vi "PH_Countdown-Counter.Calc Remaining Time.vi"(0 "i ref in":refnum<vi>, 5 "error in":errorcluster) -> (14 "i ref out":refnum<vi>, 17 "remaining Time [s]":dbl, 19 "error out":errorcluster)   [LabVIEW 2014, in "PH_Countdown-Counter.lvlib"]
uses:
  PH_Countdown-Counter.lvlib
  PH_Basics/PH_PP_Common/PH_PP_Common.PUs.ctl
  PH_Basics/PH_PP_Common/PH_PP_Common.Trigger Tags.ctl
  PH_Basics/PH_Common/PH_Common.lvlib
  CSlibraries-extern/DimLVEvent/LVDimInterface/LVDimInterface.lvlib
  PH_Basics/PH_PP_Common/PH_PP_Common.lvlib
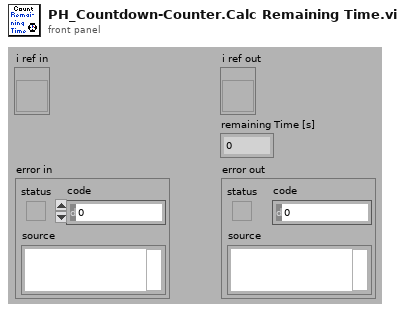
[diagram p1: front panel]
types:
  T1 = typedef "PH_Countdown-Counter.lvlib/PH_Countdown-Counter.i attribute.ctl" = cluster{"Machine Time":cluster{"Tag":string, "Wating Time [s]":dbl, "not linked?":bool}[], "Last Shot":cluster{"Tag":string, "Shot Time [s]":timestamp, "not linked?":bool}[], "Time since last Shot?":bool, "Calculation":cluster{"Time between Shots [s]":dbl, "Ref Remaining Time":refnum<vi>, "Service ID":i32, "over?":bool, "Ref Time between Shots":refnum<vi>, "Ref Set Mode":refnum<vi>}, "Sound?":bool, "Reminder":cluster{"# 1":cluster{"Pretime [s]":dbl, "Aktive?":bool, "Over?":bool}, "# 2":cluster{"Pretime [s]":dbl, "Aktive?":bool, "Over?":bool}}, "MainAmp only":cluster{"State":bool, "GUI Ref":refnum<vi>}}
  T2 = cluster{"Tag":string, "Shot Time [s]":timestamp, "not linked?":bool}[]
  T3 = cluster{"Tag":string, "Wating Time [s]":dbl, "not linked?":bool}[]
  T4 = typedef "PH_PP_Common.lvlib/PH_PP_Common.Trigger Tags.ctl" = enum16{"triggered", "fired", "Status", "Last Shot"}
  T5 = typedef "PH_PP_Common.lvlib/PH_PP_Common.PUs.ctl" = enum16{"no Info", "PA-19mm-1", "PA-19mm-2", "PA-45mm-PILC", "PA-45mm-MAIN", "MA-PU-1", "MA-PU-2", "MA-PU-3", "MA-PU-4", "MA-PU-5", "MA-PU-6", "MA-FR", "MA-PILC", "PA-45mm-DP"}
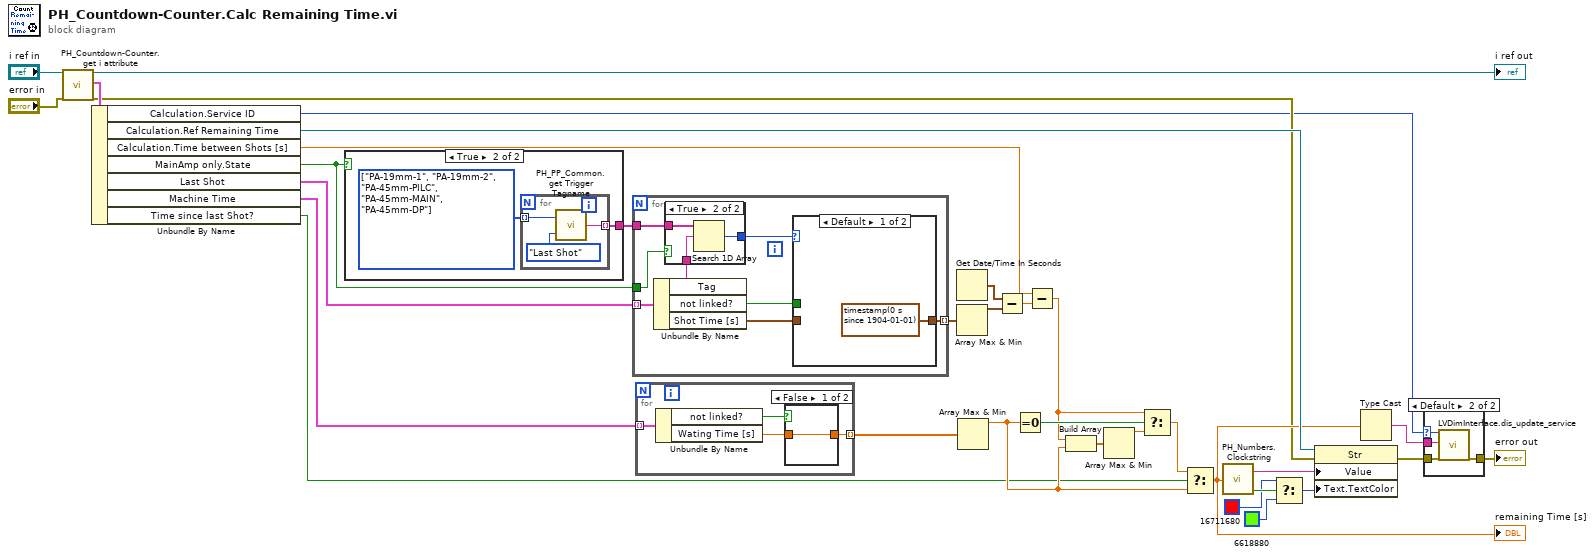
[diagram p0: block diagram]
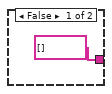
[diagram p2: hidden frame]
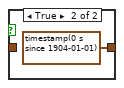
[diagram p5: hidden frame]
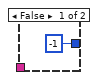
[diagram p6: hidden frame]
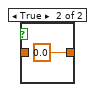
[diagram p7: hidden frame]
diagram:
  n1 = call "PH_Countdown-Counter.get i attribute.vi"("i ref in"="i ref in", "error in (no error)"="error in") -> ("i ref out"=→"i ref out":refnum<vi>, "i attribute"=w30:T1, "error out"=w6:errorcluster)  [unwired: 15 in]
  n2 = Unbundle By Name(w30) -> ("Calculation.Service ID"=w4:i32, "Calculation.Ref Remaining Time"=w16:refnum<vi>, "Calculation.Time between Shots [s]"=w24:dbl, "MainAmp only.State"=w1:bool, "Last Shot"=w3:T2, "Machine Time"=w29:T3, "Time since last Shot?"=w15:bool)
  n3 = case shown="True" w1 {
    tunnel: [string[] [] w35] -> w2
    frame False {
    }
    frame True {
      w36 = T5[] [enum."PA-19mm-1", enum."PA-19mm-2", enum."PA-45mm-PILC", enum."PA-45mm-MAIN", enum."PA-45mm-DP"] items=["no Info", "PA-19mm-1", "PA-19mm-2", "PA-45mm-PILC", "PA-45mm-MAIN", "MA-PU-1", "MA-PU-2", "MA-PU-3", "MA-PU-4", "MA-PU-5", "MA-PU-6", "MA-FR", "MA-PILC", "PA-45mm-DP"]
      n4 = for {
        tunnel: w36 -> [w38] mode=indexing
        tunnel: [w37] -> w35 mode=indexing
        n5 = call "PH_PP_Common.get Trigger Tagname.vi"("Trigger Tag"=PH_PP_Common.Trigger_Tags."Last Shot", "PU"=w38) -> ("Trigger Tagname"=w37:string)
      }
    }
  }
  n6 = for {
    tunnel: w3 -> [w47] mode=indexing
    tunnel: [w45] -> w27 mode=indexing
    tunnel: w2 -> [w43]
    tunnel: w1 -> [w41]
    n7 = Unbundle By Name(w47) -> ("Tag"=w42:string, "not linked?"=w46:bool, "Shot Time [s]"=w44:timestamp)
    n8 = case shown="True" w41 {
      tunnel: w43 -> [_ w57]
      tunnel: w42 -> [_ w56]
      tunnel: [-1 ("index of element") w55] -> w40
      frame False {
      }
      frame True {
        n9 = Search 1D Array(1D array=w57, element=w56) -> (index of element=w55:i32)  [unwired: 1 in]
      }
    }
    n10 = case shown="Default" w40 {
      tunnel: w46 -> [_ w51]
      tunnel: [timestamp(0 s since 1904-01-01) ("Shot Time [s]") w50] -> w45
      tunnel: w44 -> [_ w49]
      frame Default {
      }
      frame -1 {
        n11 = case shown="False" w51 {
          tunnel: [w52 timestamp(0 s since 1904-01-01) ("Shot Time [s]")] -> w50
          tunnel: w49 -> [w52 _]
          frame False {
          }
          frame True {
          }
        }
      }
    }
  }
  n12 = for {
    tunnel: w29 -> [w61] mode=indexing
    tunnel: [w59] -> w28 mode=indexing
    n13 = Unbundle By Name(w61) -> ("not linked?"=w60:bool, "Wating Time [s]"=w58:dbl)
    n14 = case shown="False" w60 {
      tunnel: [w62 0.0 ("Wating Time [s]")] -> w59
      tunnel: w58 -> [w62 _]
      frame False {
      }
      frame True {
      }
    }
  }
  n15 = Get Date/Time In Seconds() -> (seconds since 1Jan1904=w26:timestamp)
  n16 = Array Max & Min(array=w27) -> (max value=w25:timestamp)  [unwired: 3 out]
  n17 = Array Max & Min(array=w28) -> (max value=w19:dbl)  [unwired: 3 out]
  n18 = Subtract(x=w26, y=w25) -> (x-y=w23:dbl)
  n19 = Equal To 0?(x=w19) -> (x = 0?=w22:bool)
  n20 = Subtract(x=w24, y=w23) -> (x-y=w18:dbl)
  n21 = Build Array(w18, w19) -> (w20:dbl[])
  n22 = Array Max & Min(array=w20) -> (max value=w17:dbl)  [unwired: 3 out]
  n23 = Select(t=w18, s=w22, f=w17) -> (s? t:f=w21:dbl)
  n24 = Select(t=w21, s=w15, f=w19) -> (s? t:f=w8:dbl)
  "remaining Time [s]" <- w8
  n25 = call "PH_Numbers.Clockstring.vi"("Time [s]"=w8) -> ("Clock String"=w14:string, "<0?"=w13:bool)
  n26 = Select(t=u32 16711680 ("Color Box"), s=w13, f=u32 6618880 ("Color Box")) -> (s? t:f=w12:u32)
  n27 = property class="Str"(reference=w16, error in=w6, "Value"=w14, "Text.TextColor"=w12) -> (error out=w5:errorcluster)  [unwired: 1 out]
  n28 = Type Cast(x=w8) -> (*(type *) &x=w9:string)  [unwired: 1 in]
  n29 = case shown="Default" w4 {
    selector: w4 -> [_ w65]
    tunnel: w5 -> [w64 w68]
    tunnel: [w64 w67] -> w7
    tunnel: w9 -> [_ w66]
    frame -1 {
    }
    frame Default {
      n30 = call "LVDimInterface.dis_update_service.vi"("my_serviceID"=w65, "data"=w66, "error in (no error)"=w68) -> ("error out"=w67:errorcluster)  [unwired: 14 in, 2 out]
    }
  }
  "error out" <- w7
